vi "DecodeLookupService.vi"(3 "Response":string) -> (1 "Reply":T1(array[cluster]))   [LabVIEW 2016]
doc: "Organizes lookup service response into an array of clusters"
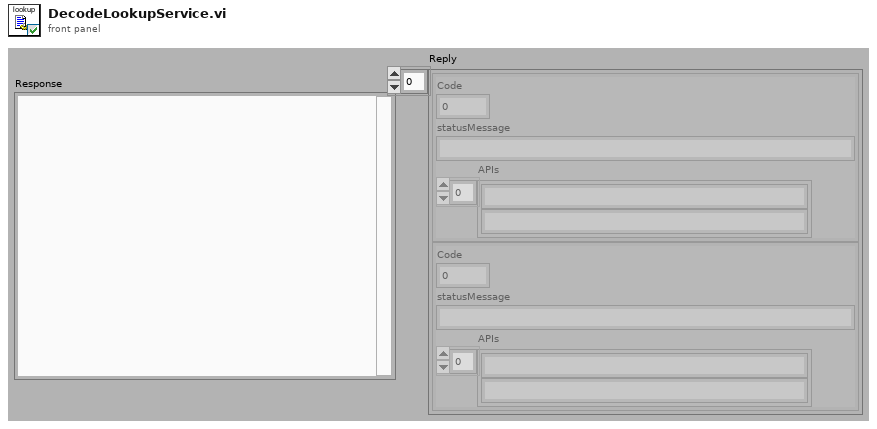
[diagram p1: front panel]
types:
  T1 = cluster{"Code":i8, "statusMessage":string, "APIs":string[]}[]
  T2 = cluster{"Code":i8, "statusMessage":string, "APIs":string[]}
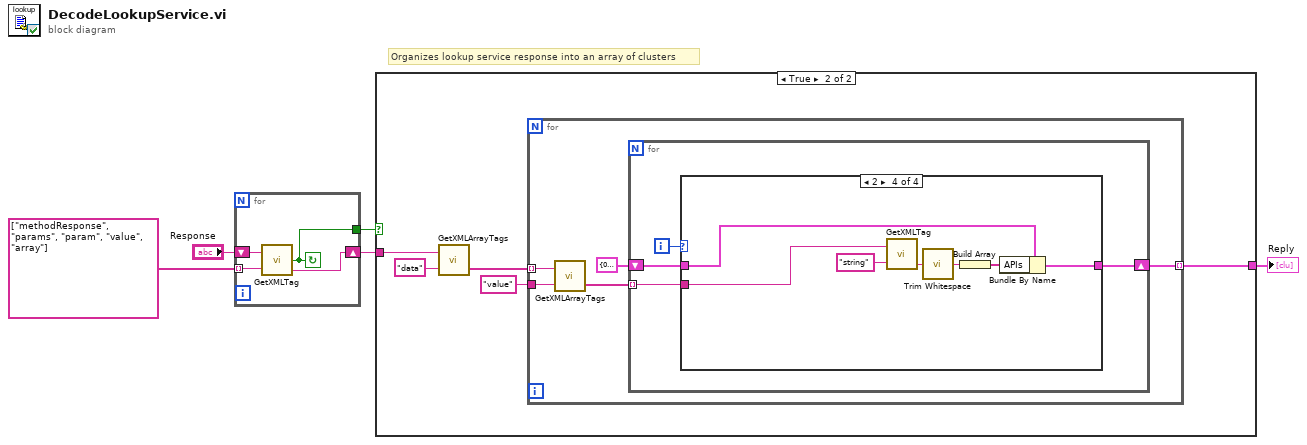
[diagram p0: block diagram]
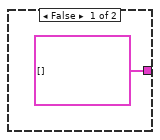
[diagram p2: hidden frame]
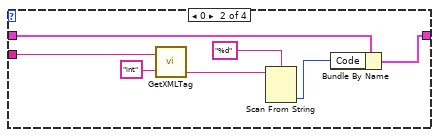
[diagram p4: hidden frame]
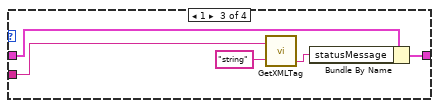
[diagram p5: hidden frame]
diagram:
  # "Organizes lookup service response into an array of clusters"
  n1 = for {
    tunnel: string[] ["methodResponse", "params", "param", "value", "array"] -> [w9] mode=indexing
    shift-right: [w7] -> w4
    shift-left: "Response" -> [w8]
    tunnel: [w6] -> w2
    stop <- w6 continue-if-true
    n2 = call "GetXMLTag.vi"("Tag"=w9, "String"=w8) -> ("Value"=w7:string, "Exists?"=w6:bool)  [unwired: 1 out]
  }
  n3 = case shown="True" w2 {
    tunnel: w4 -> [_ w12]
    tunnel: [T1 [] w11] -> w3
    frame False {
    }
    frame True {
      n4 = call "GetXMLArrayTags.vi"("ArrayTag"="data", "String"=w12) -> ("Array"=w14:string[])  [unwired: 1 out]
      n5 = for {
        tunnel: w14 -> [w20] mode=indexing
        tunnel: "value" -> [w19]
        tunnel: [w16] -> w11 mode=indexing
        n6 = call "GetXMLArrayTags.vi"("ArrayTag"=w19, "String"=w20) -> ("Array"=w18:string[])  [unwired: 1 out]
        n7 = for {
          tunnel: w18 -> [w24] mode=indexing
          shift-right: [w21] -> w16
          shift-left: T2 {"Code"=0, "statusMessage"="", "APIs"=[]} ("Parameters") -> [w22]
          i -> [w23]
          n8 = case shown="2" w23 {
            tunnel: w24 -> [_ w31 w36 w41]
            tunnel: w22 -> [w25 w28 w35 w44]
            tunnel: [w25 w26 w34 w43] -> w21
            frame Default {
            }
            frame 0 {
              n9 = call "GetXMLTag.vi"("Tag"="int", "String"=w31) -> ("Value"=w30:string)  [unwired: 2 out]
              n10 = Scan From String(format string="%d", input string=w30) -> (output 1=w27:i32)  [unwired: 3 in, 3 out]
              n11 = Bundle By Name(cluster=w28, "Code"=w27) -> (w26:T2)
            }
            frame 1 {
              n12 = call "GetXMLTag.vi"("Tag"="string", "String"=w36) -> ("Value"=w33:string)  [unwired: 2 out]
              n13 = Bundle By Name(cluster=w35, "statusMessage"=w33) -> (w34:T2)
            }
            frame 2 {
              n14 = call "GetXMLTag.vi"("Tag"="string", "String"=w41) -> ("Value"=w40:string)  [unwired: 2 out]
              n15 = call "Trim Whitespace.vi"("string"=w40) -> ("trimmed string"=w38:string)  [unwired: 1 in]
              n16 = Build Array(w38) -> (w39:string[])
              n17 = Bundle By Name(cluster=w44, "APIs"=w39) -> (w43:T2)
            }
          }
        }
      }
    }
  }
  "Reply" <- w3
